vi "MainWindow.vi"(10 "queueName":string="PV_script", 11 "Path":path=path "/Users/crogers/GitHub/ME35_21/PythonIDE/Codes/Examples/SPIKE/Sensors.py") -> ()   [LabVIEW 2022 SP3]
panel:
  out "Text.Scroll Position":u32
  in  "Python Code":string
  out "Line #":string
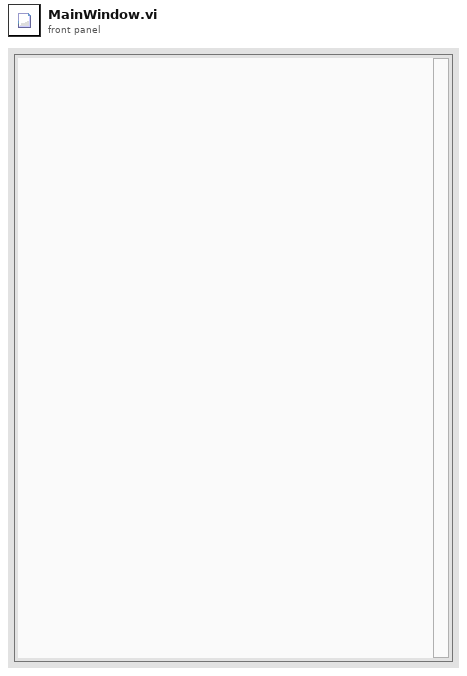
[diagram p1: front panel]
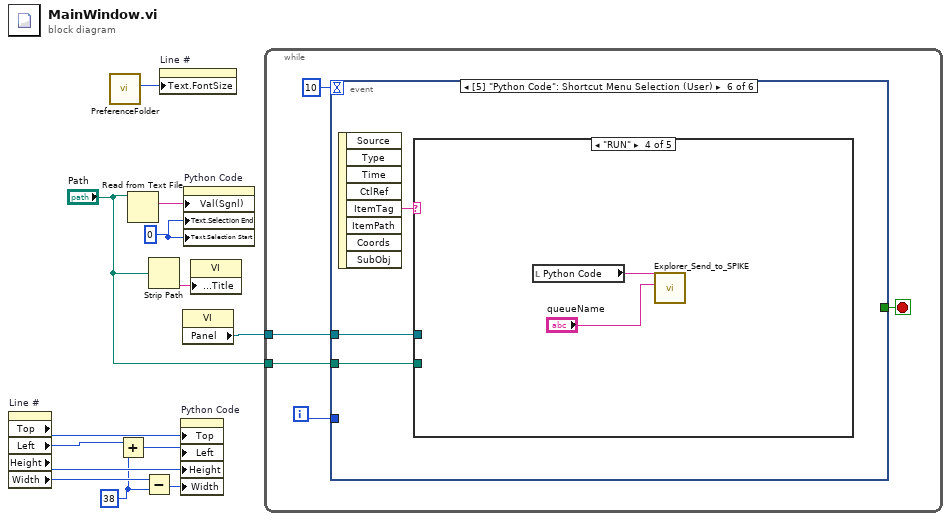
[diagram p0: block diagram]
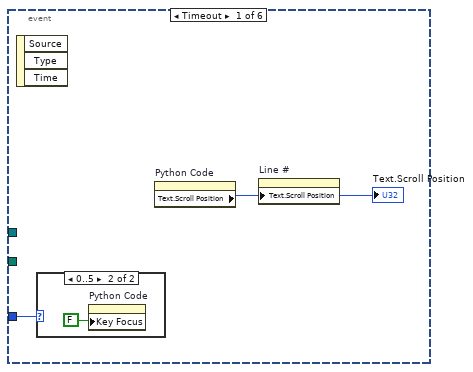
[diagram p2: hidden frame]
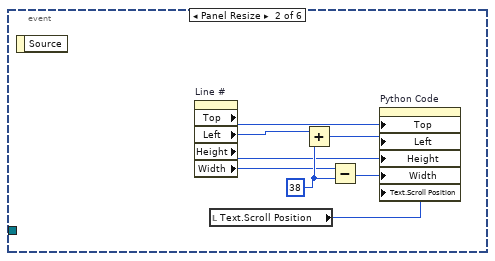
[diagram p4: hidden frame]
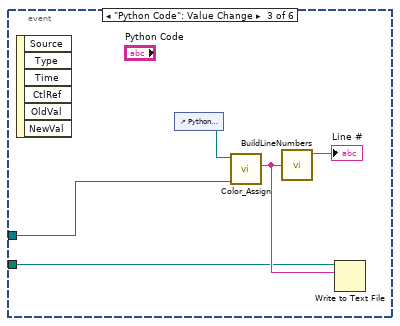
[diagram p5: hidden frame]
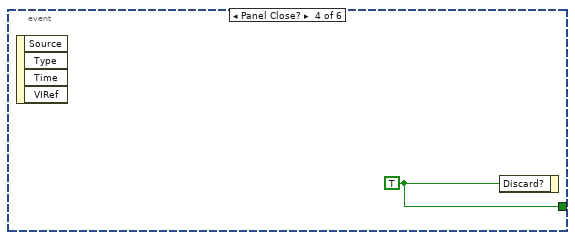
[diagram p6: hidden frame]
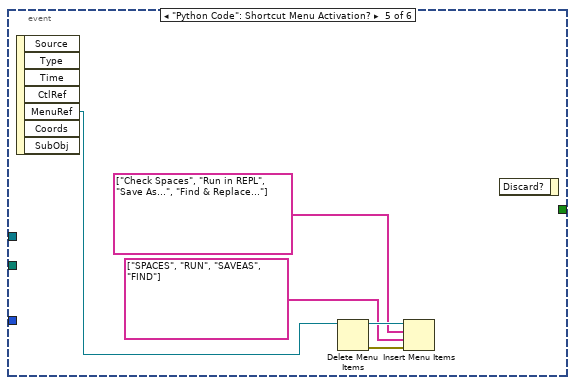
[diagram p7: hidden frame]
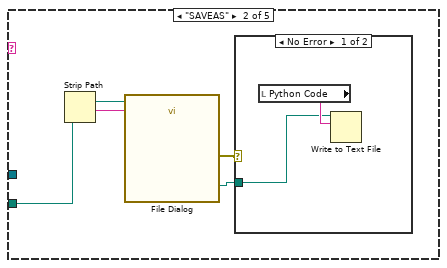
[diagram p9: hidden frame]
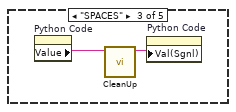
[diagram p11: hidden frame]
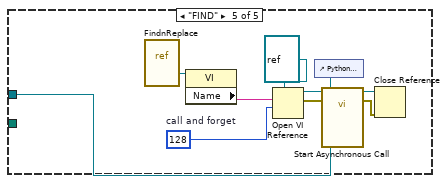
[diagram p12: hidden frame]
diagram:
  w3 = u32 0 ("Text.Selection:End")
  w7 = 38 ("y")
  n1 = property on="Line #" class="Str"() -> ("Top"=w10:i32, "Left"=w8:i32, "Height"=w11:u32, "Width"=w12:u32)  [unwired: 2 in, 2 out]
  n2 = call "PreferenceFolder.vi"() -> ("FontSize"=w2:u8)  [unwired: 4 in, 7 out]
  n3 = Add(x=w8, y=w7) -> (x+y=w9:i32)
  n4 = Read from Text File(file (use dialog)="Path") -> (text=w5:string)  [unwired: 3 in, 3 out]
  n5 = Subtract(x=w12, y=w7) -> (x-y=w13:u32)
  n6 = Strip Path(path="Path") -> (name=w6:string)  [unwired: 1 out]
  n7 = property on="Line #" class="Str"("Text.FontSize"=w2) -> ()  [unwired: 2 in, 2 out]
  n8 = property on="Python Code" class="Str"("Top"=w10, "Left"=w9, "Height"=w11, "Width"=w13) -> ()  [unwired: 2 in, 2 out]
  n9 = property class="VI"() -> ("Panel"=w1:refnum<vi>)  [unwired: 2 in, 2 out]
  n10 = property on="Python Code" class="Str"("Val(Sgnl)"=w5, "Text.Selection End"=w3, "Text.Selection Start"=w3) -> ()  [unwired: 2 in, 2 out]
  n11 = property class="VI"("Front Panel.Title"=w6) -> ()  [unwired: 2 in, 2 out]
  n12 = while {
    tunnel: "Path" -> [w16]
    tunnel: w1 -> [w14]
    i -> [w15]
    stop <- w18 stop-if-true
    n13 = event shown="[5] \"Python Code\": Shortcut Menu Selection (User)" {
      selector: _ -> [_ _ _ _ _ _]
      dyn-events: _ -> [_ _ _ _ _ _]
      timeout: 10 -> [_ _ _ _ _ _]
      tunnel: [_ _ _ w35 _ _] -> w18
      tunnel: w16 -> [_ _ w31 _ _ w43]
      tunnel: w15 -> [w19 _ _ _ _ _]
      tunnel: w14 -> [_ _ w30 _ _ w41]
      event Timeout {
        n14 = event-data() -> ()  [unwired: 1 in, 3 out]
        n15 = case shown="0..5" w19 {
          frame Default {
          }
          frame 0..5 {
            n16 = property on="Python Code" class="Str"("Key Focus"=FALSE) -> ()  [unwired: 2 in, 2 out]
          }
        }
        n17 = property on="Python Code" class="Str"() -> ("Text.Scroll Position"=w20:u32)  [unwired: 2 in, 2 out]
        "Text.Scroll Position" <- w20
        n18 = property on="Line #" class="Str"("Text.Scroll Position"=w20) -> ()  [unwired: 2 in, 2 out]
      }
      event Panel Resize {
        w29 = 38 ("y")
        n19 = event-data() -> ()  [unwired: 1 in, 1 out]
        n20 = property on="Line #" class="Str"() -> ("Top"=w26:i32, "Left"=w28:i32, "Height"=w25:u32, "Width"=w24:u32)  [unwired: 2 in, 2 out]
        n21 = local read "Text.Scroll Position"() -> (w22:u32)
        n22 = Add(x=w28, y=w29) -> (x+y=w27:i32)
        n23 = Subtract(x=w24, y=w29) -> (x-y=w23:u32)
        n24 = property on="Python Code" class="Str"("Top"=w26, "Left"=w27, "Height"=w25, "Width"=w23, "Text.Scroll Position"=w22) -> ()  [unwired: 2 in, 2 out]
      }
      event "Python Code": Value Change {
        n25 = event-data() -> ()  [unwired: 1 in, 6 out]
        n26 = control-ref of="Python Code"() -> (w34:refnum<vi>)
        n27 = call "Color_Assign.vi"("Front Panel"=w30, "Code"=w34) -> ("Value"=w32:string)  [unwired: 9 in]
        n28 = call "BuildLineNumbers.vi"("Python Code"=w32) -> ("String"=→"Line #":string)  [unwired: 10 in]
        n29 = Write to Text File(file (use dialog)=w31, text=w32) -> ()  [unwired: 2 in, 3 out]
      }
      event Panel Close? {
        w35 = TRUE ("Discard?")
        n30 = event-data() -> ()  [unwired: 1 in, 4 out]
        n31 = event-data("Discard?"=w35) -> ()  [unwired: 1 in, 1 out]
      }
      event "Python Code": Shortcut Menu Activation? {
        n32 = event-data() -> ("MenuRef"=w36:refnum<k9>)  [unwired: 1 in, 6 out]
        n33 = Delete Menu Items(9:w36) -> (0:w40:errorcluster, 3:w39:refnum<k9>)  [unwired: 3 in]
        n34 = Insert Menu Items(6:w40, 7:string[] ["SPACES", "RUN", "SAVEAS", "FIND"], 8:string[] ["Check Spaces", "Run in REPL", "Save As...", "Find & Replace..."] ("L10n_Parent Menus"), 9:w39) -> ()  [unwired: 2 in, 3 out]
        n35 = event-data() -> ()  [unwired: 2 in, 1 out]
      }
      event "Python Code": Shortcut Menu Selection (User) {
        n36 = event-data() -> ("ItemTag"=w42:string)  [unwired: 1 in, 7 out]
        n37 = case shown="\"RUN\"" w42 {
          tunnel: w43 -> [_ w44 _ _ _]
          tunnel: w41 -> [_ _ _ _ w55]
          frame Default {
          }
          frame "SAVEAS" {
            n38 = Strip Path(path=w44) -> (stripped path=w46:path, name=w45:string)
            n39 = call "File Dialog"("start path"=w46, "default name"=w45) -> ("selected path"=w47:path, "error out"=w48:errorcluster)  [unwired: 10 in, 2 out]
            n40 = case shown="No Error" w48 {
              tunnel: w47 -> [w49 _]
              frame No Error {
                n41 = local read "Python Code"() -> (w50:string)
                n42 = Write to Text File(file (use dialog)=w49, text=w50) -> ()  [unwired: 2 in, 3 out]
              }
              frame Error {
              }
            }
          }
          frame "SPACES" {
            n43 = property on="Python Code" class="Str"() -> ("Value"=w51:string)  [unwired: 2 in, 2 out]
            n44 = call "CleanUp.vi"("Python Code"=w51) -> ("spreadsheet string"=w52:string)  [unwired: 10 in]
            n45 = property on="Python Code" class="Str"("Val(Sgnl)"=w52) -> ()  [unwired: 2 in, 2 out]
          }
          frame "RUN" {
            n46 = local read "Python Code"() -> (w54:string)
            n47 = call "Explorer_Send_to_SPIKE.vi"("queueName"="queueName", "python"=w54) -> ()  [unwired: 9 in, 1 out]
          }
          frame "FIND" {
            w57 = 128  # call and forget
            n48 = vi-ref "FindnReplace.vi"() -> (w62:refnum<vi>)
            n49 = property class="VI"(reference=w62) -> ("Name"=w63:string)  [unwired: 1 in, 2 out]
            n50 = Open VI Reference(type specifier VI Refnum (for type only)=refnum<vi> refnum, vi path=w63, options=w57) -> (vi reference=w64:refnum<vi>, error out=w59:errorcluster)  [unwired: 3 in]
            n51 = control-ref of="Python Code"() -> (w56:refnum<vi>)
            n52 = call-by-ref "Start Asynchronous Call"(reference=w64, error in=w59, "Front Panel"=w55, "Python Code"=w56) -> (reference out=w60:refnum<vi>, error out=w61:errorcluster)  [unwired: 10 in]
            n53 = Close Reference(reference=w60, error in (no error)=w61) -> ()  [unwired: 1 out]
          }
        }
      }
    }
  }
